vi "PSO_UpdateGbestParticle.vi"(9 "Gbest Fitness":dbl, 10 "Gbest Particle":i32[](array[numeric]), 11 "Population in":T1) -> (1 "Fitness":dbl, 2 "Solution":i32[](array[numeric]), 3 "Population out":T1)   [LabVIEW 2016, in "Optimal Frequency Bands Search.lvlib" / "ParticleSwarm.lvlib"]
doc: "Найти частицу с лучшими координатами (с учетом значения функции приспособленности)"
uses:
  ParticleSwarm.lvlib
  PSO_tPopulation.ctl
panel:
  # "This VI is a part of BCI Design library, http://www.ru-bci.org \nCopyright © 2020, Sotnikov Peter, All rights reserved. License: CC BY-NC 4.0"
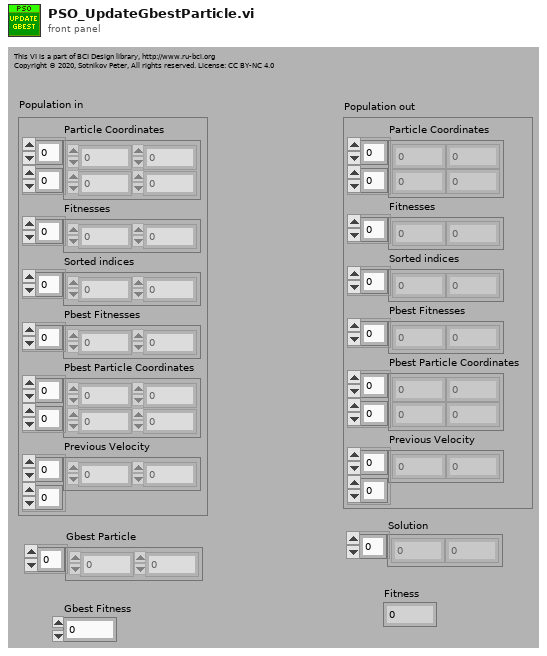
[diagram p1: front panel]
types:
  T1 = typedef "Optimal Frequency Bands Search.lvlib/ParticleSwarm.lvlib/PSO_tPopulation.ctl" = cluster{"Particle Coordinates":i32[][], "Fitnesses":dbl[], "Sorted indices":i32[], "Pbest Fitnesses":dbl[], "Pbest Particle Coordinates":i32[][], "Previous Velocity":dbl[][]}
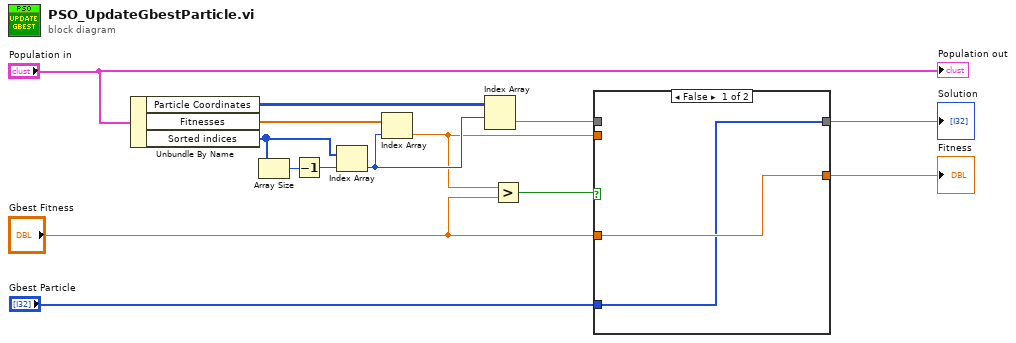
[diagram p0: block diagram]
diagram:
  n1 = Unbundle By Name("Population in") -> ("Particle Coordinates"=w9:i32[][], "Fitnesses"=w11:dbl[], "Sorted indices"=w12:i32[])
  n2 = Array Size(array=w12) -> (size(s)=w14:i32)
  n3 = Decrement(x=w14) -> (x-1=w13:i32)
  n4 = Index Array(array=w12, index=w13) -> (element=w8:i32)
  n5 = Index Array(array=w11, index=w8) -> (element=w3:dbl)
  n6 = Index Array "Index Array"(array=w9, index (row)=w8) -> (element=w7:i32[])  [unwired: 1 in]
  n7 = Greater?(x=w3, y="Gbest Fitness") -> (0:w6:bool)
  n8 = case shown="False" w6 {
    tunnel: w7 -> [_ w18]
    tunnel: "Gbest Particle" -> [w15 _]
    tunnel: "Gbest Fitness" -> [w16 _]
    tunnel: w3 -> [_ w17]
    tunnel: [w15 w18] -> w2
    tunnel: [w16 w17] -> w1
    frame False {
    }
    frame True {
    }
  }
  "Solution" <- w2
  "Fitness" <- w1
  "Population out" <- "Population in"
